vi "Periodic Tasks.vi"(8 "error in":errorcluster) -> ()   [LabVIEW 2018]
doc: "This VI runs in parallel to other tasks. It can contain as many user-defined periodic loops as you need. These can carry out PID or other sorts of timed response."
uses:
  <vilib>/Rock Robotics/WPI/Joystick/WPI_JoystickDevRef.ctl
  <vilib>/Rock Robotics/WPI/Joystick/WPI_JoystickDeviceEnum.ctl
  <vilib>/Rock Robotics/WPI/Utilities/WPI_GetSetVariantRefNum.vi
  Robot Global Data.vi
panel:
  out "Drive Joy Loop":u32=14
  # "Loop Speeds"
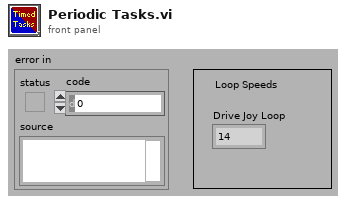
[diagram p1: front panel]
types:
  T1 = enum16{"Two Logitec Extremes", "Dual Action Logitec", "Interlink"}
  T2 = typedef "WPI_JoystickDevRef.ctl" = cluster{"Device":T3}
  T3 = typedef "WPI_JoystickDeviceEnum.ctl" = enum16{"USB 0", "USB 1", "USB 2", "USB 3", "USB 4", "USB 5"}
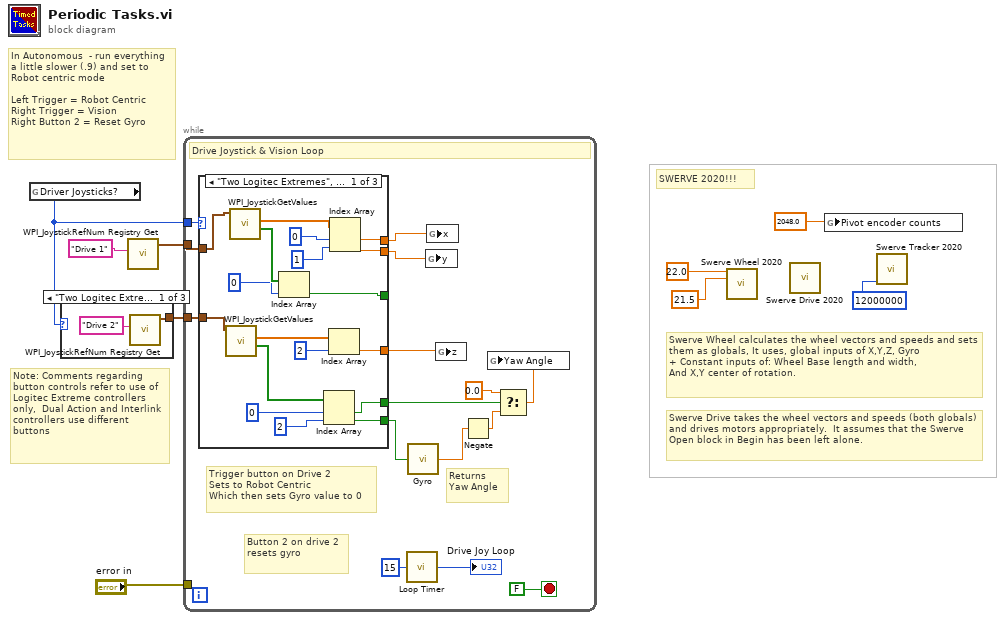
[diagram p0: block diagram]
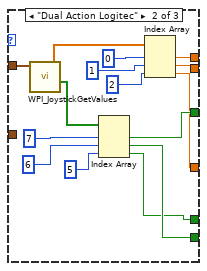
[diagram p2: hidden frame]
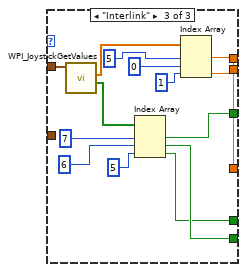
[diagram p3: hidden frame]
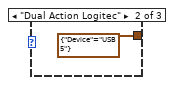
[diagram p4: hidden frame]
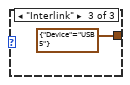
[diagram p5: hidden frame]
diagram:
  # "Note: Comments regarding button controls refer to use of Logitec Extreme controllers only,  Dual Action and Interlink controllers use different buttons"
  # "Swerve Drive takes the wheel vectors and speeds (both globals) and drives motors appropriately.  It assumes that the Swerve Open block in Begin has been left alone."
  # "Swerve Wheel calculates the wheel vectors and speeds and sets them as globals, It uses, global inputs of X,Y,Z, Gyro\n+ Constant inputs of: Wheel Base length and width,\nAnd X,Y center of rotation."
  # "In Autonomous  - run everything a little slower (.9) and set to Robot centric mode\n\nLeft Trigger = Robot Centric\nRight Trigger = Vision\nRight Button 2 = Reset Gyro"
  # "SWERVE 2020!!!"
  n1 = global read "Robot Global Data.vi" "Driver Joysticks?"() -> (w4:T1)
  n2 = case shown="\"Two Logitec Extremes\"" w4 {
    tunnel: [w10 T2 {"Device"=enum."USB 5"} ("JoystickDevRef") T2 {"Device"=enum."USB 5"} ("JoystickDevRef")] -> w7
    frame "Two Logitec Extremes" {
      n3 = call <vilib>:"WPI_JoystickRefNum Registry Get.vi"("refnum name"="Drive 2") -> ("JoystickDevRef"=w10:T2)  [unwired: 9 in, 1 out]
    }
    frame "Dual Action Logitec" {
    }
    frame "Interlink" {
    }
  }
  n4 = call <vilib>:"WPI_JoystickRefNum Registry Get.vi"("refnum name"="Drive 1") -> ("JoystickDevRef"=w9:T2)  [unwired: 9 in, 1 out]
  n5 = while {
    tunnel: w9 -> [w28]
    tunnel: w7 -> [w27]
    tunnel: w4 -> [w25]
    tunnel: "error in" -> [_]
    stop <- FALSE stop-if-true
    # "Returns Yaw Angle"
    # "Trigger button on Drive 2 \nSets to Robot Centric\nWhich then sets Gyro value to 0"
    # "Button 2 on drive 2 resets gyro"
    # "Drive Joystick & Vision Loop"
    n6 = case shown="\"Two Logitec Extremes\", Default" w25 {
      tunnel: w28 -> [w42 w61 w65]
      tunnel: [w32 w50 w70] -> w20
      tunnel: [w40 w52 w69] -> w18
      tunnel: [w39 w51 w67] -> w19
      tunnel: [w31 w47 w62] -> w15
      tunnel: [w38 w56 w66] -> _
      tunnel: w27 -> [w33 _ _]
      tunnel: [w30 w49 w64] -> w22
      frame "Two Logitec Extremes", Default {
        n7 = call <vilib>:"WPI_JoystickGetValues.vi"("JoystickDevRef"=w33) -> ("Buttons"=w37:bool[], "Axes"=w34:dbl[])  [unwired: 6 in, 3 out]
        n8 = call <vilib>:"WPI_JoystickGetValues.vi"("JoystickDevRef"=w42) -> ("Buttons"=w46:bool[], "Axes"=w41:dbl[])  [unwired: 6 in, 3 out]
        n9 = Index Array(array=w46, index=0) -> (element=w38:bool)
        n10 = Index Array(array=w37, index #1=0 ("index"), index #2=2 ("index")) -> (element #1=w31:bool, element #2=w30:bool)
        n11 = Index Array(array=w34, index=2) -> (element=w32:dbl)
        n12 = Index Array(array=w41, index #1=0 ("index"), index #2=1 ("index")) -> (element #1=w40:dbl, element #2=w39:dbl)
      }
      frame "Dual Action Logitec" {
        n13 = call <vilib>:"WPI_JoystickGetValues.vi"("JoystickDevRef"=w61) -> ("Buttons"=w59:bool[], "Axes"=w60:dbl[])  [unwired: 6 in, 3 out]
        n14 = Index Array(array=w59, index #1=7 ("index"), index #2=6 ("index"), index #3=5 ("index")) -> (element #1=w56:bool, element #2=w49:bool, element #3=w47:bool)
        n15 = Index Array(array=w60, index #1=0 ("index"), index #2=1 ("index"), index #3=2 ("index")) -> (element #1=w52:dbl, element #2=w51:dbl, element #3=w50:dbl)
      }
      frame "Interlink" {
        n16 = call <vilib>:"WPI_JoystickGetValues.vi"("JoystickDevRef"=w65) -> ("Buttons"=w76:bool[], "Axes"=w68:dbl[])  [unwired: 6 in, 3 out]
        n17 = Index Array(array=w76, index #1=7 ("index"), index #2=6 ("index"), index #3=5 ("index")) -> (element #1=w66:bool, element #2=w64:bool, element #3=w62:bool)
        n18 = Index Array(array=w68, index #1=5 ("index"), index #2=0 ("index"), index #3=1 ("index")) -> (element #1=w70:dbl, element #2=w69:dbl, element #3=w67:dbl)
      }
    }
    n19 = call "Loop Timer.vi"("Wait time"=u32 15 ("millisecond multiple")) -> ("Loop Time"=→"Drive Joy Loop":u32)
    n20 = call "Gyro.vi"("Reset Gyro"=w22) -> ("Yaw Angle"=w21:dbl)
    n21 = global write "Robot Global Data.vi" "y"(w19) -> ()
    n22 = global write "Robot Global Data.vi" "x"(w18) -> ()
    n23 = global write "Robot Global Data.vi" "z"(w20) -> ()
    n24 = Negate(x=w21) -> (-x=w14:dbl)
    n25 = Select(t=0.0, s=w15, f=w14) -> (s? t:f=w16:dbl)
    n26 = global write "Robot Global Data.vi" "Yaw Angle"(w16) -> ()
  }
  n27 = call "Swerve Wheel 2020.vi"("Wheelbase Length"=22.0, "Wheelbase Width"=21.5) -> ()  [unwired: 14 in]
  n28 = call "Swerve Drive 2020.vi"() -> ()  [unwired: 4 in]
  n29 = global write "Robot Global Data.vi" "Pivot encoder counts"(2048.0 ("Pivot encoder counts")) -> ()
  n30 = call "Swerve Tracker 2020.vi"("Calibration Constant"=12000000 ("Numeric")) -> ()  [unwired: 15 in]
